vi "Element Init.vi"(7 "VolatusAPI":refnum<class "VolatusAPI.lvclass">, 8 "error in (no error)":errorcluster, 10 "JSON":string, 11 "BooleanIndicator in":refnum<class "BooleanIndicator.lvclass">) -> (0 "error out":errorcluster, 3 "BooleanIndicator out":refnum<class "BooleanIndicator.lvclass">)   [LabVIEW 2020, in "VolatusGUIElements.lvlib" / "BooleanIndicator.lvclass"]
uses:
  BooleanIndicator.lvclass
  Volatus/VolatusAPI/VolatusAPI.lvclass
  JSON.ctl
  lv-vecto/Vecto/Group DBL/Group DBL.lvclass
  C:/dev/lv20CE/relink/lv-vecto/Vecto/Group/Group.lvclass
  BooleanIndicator.lvclass/BooleanIndicator.ctl
  7089c811-0f34-4f74-ae8a-ef1214646352.vi
  <vilib>/JDP Science/JSONtext/JSON text to Variant.vi
  <vilib>/JDP Science/JSONtext/LVClass Serializer/JSONtext LVClass Serializer.lvclass
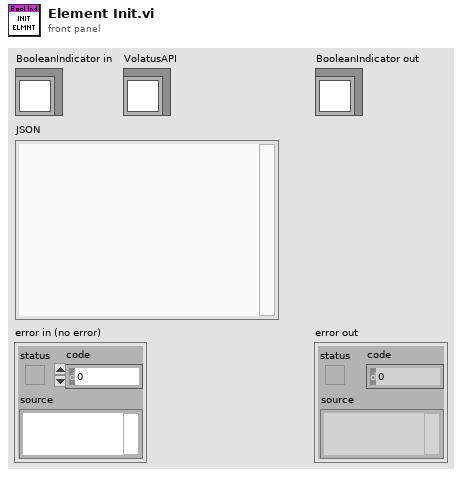
[diagram p1: front panel]
types:
  T1 = typedef "VolatusGUIElements.lvlib/BooleanIndicator.lvclass/JSON.ctl" = cluster{"Channel":string}
  T2 = typedef "VectoConfig.lvlib/Channel Info.ctl" = cluster{"Name":string, "Group":string, "Owning Node":string, "Owning Task":string, "Resource":string}
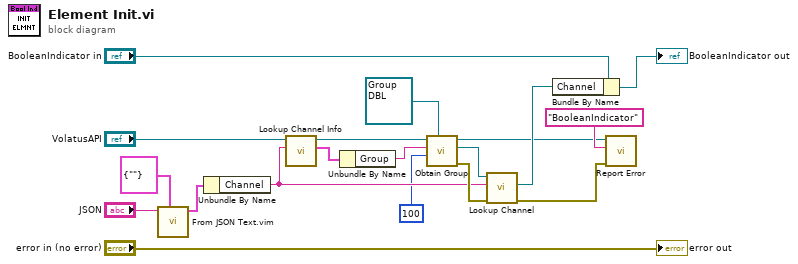
[diagram p0: block diagram]
diagram:
  n1 = call "From JSON Text.vim"("Data Type and Default Value"=T1 {"Channel"=""} ("JSON"), "JSON"="JSON") -> ("Data out"=w8:T1)  [unwired: 8 in, 1 out]
  n2 = Unbundle By Name(w8) -> ("Channel"=w7:string)
  n3 = call "Lookup Channel Info.vi"("Channel Name"=w7, "VolatusAPI in"="VolatusAPI") -> ("Channel Info"=w11:T2, "VolatusAPI out"=w12:refnum<class "VolatusAPI.lvclass">)  [unwired: 6 in, 2 out]
  n4 = Unbundle By Name(w11) -> ("Group"=w10:string)
  n5 = call "Obtain Group.vi"("Group Type (Abstract)"=refnum<class "Group DBL.lvclass"> refnum ("Group in"), "Timeout ms (5000)"=u32 100, "Group Name"=w10, "VolatusAPI in"=w12) -> ("error out"=w15:errorcluster, "Group"=w13:refnum<class "Group DBL.lvclass">, "VolatusAPI out"=w3:refnum<class "VolatusAPI.lvclass">)  [unwired: 5 in]
  n6 = call "Lookup Channel.vi"("error in (no error)"=w15, "Channel Name"=w7, "Group in"=w13) -> ("error out"=w2:errorcluster, "Channel"=w5:refnum<class "Channel DBL.lvclass">)  [unwired: 6 in, 1 out]
  n7 = Bundle By Name(cluster="BooleanIndicator in", "Channel"=w5) -> (→"BooleanIndicator out":refnum<class "BooleanIndicator.lvclass">)
  n8 = call "Report Error.vi"("error in (no error)"=w2, "Context"="BooleanIndicator", "VolatusAPI in"=w3) -> ()  [unwired: 7 in, 2 out]
  "error out" <- "error in (no error)"
